vi "GenCM-Set Slot Controls.vi"(0 "connector types":T1[](array[typedef]), 7 "Slot Num":u32[](array[numeric]), 9 "slot ctl refs":refnum<vi>[](array[refnum]), 11 "error in (no error)":errorcluster, 12 "Trigger Slot":i32) -> (4 "min slot":u32, 10 "slot ctl refs out":refnum<vi>[](array[refnum]), 15 "error out":errorcluster)   [LabVIEW 2015]
uses:
  Type Defs/PXISlot XControl/Connector Type.ctl
  Type Defs/General PXISlot XControl/PXISlotGP.xctl
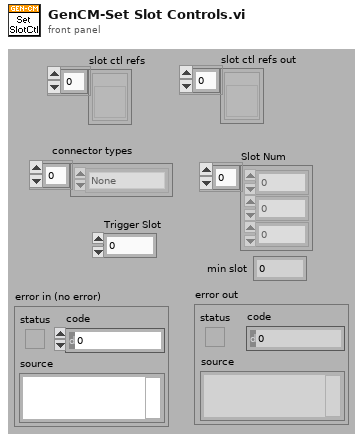
[diagram p1: front panel]
types:
  T1 = typedef "Connector Type.ctl" = enum16{"None", "PXI-4461", "BNC-2110", "BNC-2090"}
  T2 = cluster{"Output sources":string[], "Input sources":string[]}
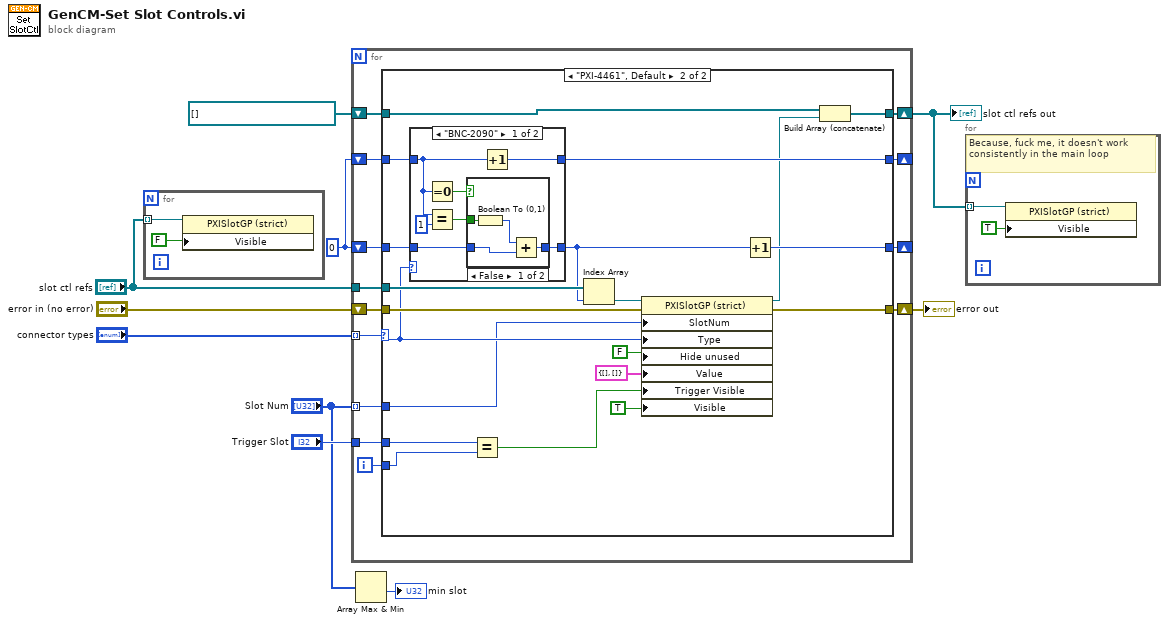
[diagram p0: block diagram]
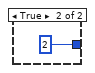
[diagram p3: hidden frame]
diagram:
  w5 = 0
  n1 = for {
    tunnel: "slot ctl refs" -> [w12] mode=indexing
    n2 = property class="PXISlotGP (strict)"(reference=w12, "Visible"=FALSE) -> ()  [unwired: 1 in, 2 out]
  }
  n3 = for {
    tunnel: "slot ctl refs" -> [w23]
    shift-right: [w24] -> w8
    shift-left: "error in (no error)" -> [w25]
    tunnel: "connector types" -> [w20] mode=indexing
    shift-right: [w21] -> _
    shift-left: w5 -> [w22]
    shift-right: [w19] -> w3
    shift-left: refnum<vi>[] [] -> [w18]
    shift-right: [w15] -> _
    shift-left: w5 -> [w16]
    tunnel: "Trigger Slot" -> [w14]
    tunnel: "Slot Num" -> [w13] mode=indexing
    i -> [w17]
    n4 = case shown="\"PXI-4461\", Default" w20 {
      selector: w20 -> [_ w35]
      tunnel: w25 -> [w28 w49]
      tunnel: [w28 w48] -> w24
      tunnel: w23 -> [_ w46]
      tunnel: w22 -> [w29 w45]
      tunnel: [w29 w44] -> w21
      tunnel: [w27 w41] -> w19
      tunnel: w18 -> [w27 w40]
      tunnel: w17 -> [_ w33]
      tunnel: w16 -> [w26 w39]
      tunnel: [w26 w38] -> w15
      tunnel: w14 -> [_ w32]
      tunnel: w13 -> [_ w34]
      frame "None" {
      }
      frame "PXI-4461", Default {
        n5 = case shown="\"BNC-2090\"" w35 {
          tunnel: w45 -> [w56 w63]
          tunnel: [w55 w63] -> w43
          tunnel: w39 -> [w51 w62]
          tunnel: [w53 w62] -> w38
          frame "BNC-2090" {
            n6 = Equal To 0?(x=w51) -> (x = 0?=w54:bool)
            n7 = Equal?(x=w51, y=1) -> (x = y?=w52:bool)
            n8 = case shown="False" w54 {
              tunnel: w56 -> [w60 _]
              tunnel: [w59 2] -> w55
              tunnel: w52 -> [w57 _]
              frame False {
                n9 = Boolean To (0,1)(Boolean=w57) -> (0, 1=w58:i16)
                n10 = Add(x=w58, y=w60) -> (x+y=w59:i32)
              }
              frame True {
              }
            }
            n11 = Increment(x=w51) -> (x+1=w53:i32)
          }
          frame "PXI-4461", Default {
          }
        }
        n12 = Equal?(x=w32, y=w33) -> (x = y?=w37:bool)
        n13 = Index Array(array=w46, index=w43) -> (element=w42:refnum<vi>)
        n14 = property class="PXISlotGP (strict)"(reference=w42, error in=w49, "SlotNum"=w34, "Type"=w35, "Hide unused"=FALSE, "Value"=T2 {"Output sources"=[], "Input sources"=[]}, "Trigger Visible"=w37, "Visible"=TRUE) -> (reference out=w31:refnum<vi>, error out=w48:errorcluster)
        n15 = Increment(x=w43) -> (x+1=w44:i32)
        n16 = Build Array (concatenate)(w40, w31) -> (w41:refnum<vi>[])
      }
    }
  }
  "error out" <- w8
  "slot ctl refs out" <- w3
  n17 = Array Max & Min(array="Slot Num") -> (min value=→"min slot":u32)  [unwired: 3 out]
  n18 = for {
    tunnel: w3 -> [w65] mode=indexing
    # "Because, fuck me, it doesn't work consistently in the main loop"
    n19 = property class="PXISlotGP (strict)"(reference=w65, "Visible"=TRUE) -> ()  [unwired: 1 in, 2 out]
  }
